vi "Create.vi"(8 "error in (no error)":errorcluster, 11 "Client in":refnum<class "Client.lvclass">) -> (0 "error out":errorcluster, 3 "Client out":refnum<class "Client.lvclass">)   [LabVIEW 2020, in "Client.lvlib" / "Client.lvclass"]
uses:
  Client.lvclass
  Client.lvclass/Client.ctl
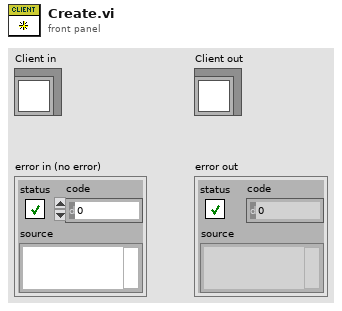
[diagram p1: front panel]
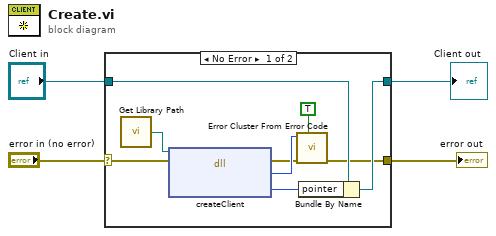
[diagram p0: block diagram]
diagram:
  n1 = case shown="No Error" "error in (no error)" {
    selector: "error in (no error)" -> [w11 w15]
    tunnel: [w8 w15] -> w3
    tunnel: [w12 w14] -> w1
    tunnel: "Client in" -> [w13 w14]
    frame No Error {
      n2 = call "Get Library Path.vi"() -> ("Path"=w7:path)  [unwired: 1 in]
      n3 = dll-call lib="?" fn="createClient"(path in=w7, error in=w11) -> (error out=w9:errorcluster, "ret_code"=w10:i32, "client"=w6:i64)  [unwired: 2 in, 1 out]
      n4 = call <vilib>:"Error Cluster From Error Code.vi"("show call chain? (False)"=TRUE, "error in (no error)"=w9, "error code (0)"=w10) -> ("error out"=w8:errorcluster)  [unwired: 6 in]
      n5 = Bundle By Name(cluster=w13, "pointer"=w6) -> (w12:refnum<class "Client.lvclass">)
    }
    frame Error {
    }
  }
  "error out" <- w3
  "Client out" <- w1
